vi "value to ring (PortType).vi"(11 "value":string) -> (3 "PortType":enum16{"FDX_UDP_SAMPLING", "FDX_UDP_QUEUING"}(ring))   [LabVIEW 2020, in "AIM ARINC 664 Import.lvlib"]
uses:
  AIM ARINC 664 Import.lvlib
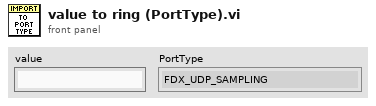
[diagram p1: front panel]
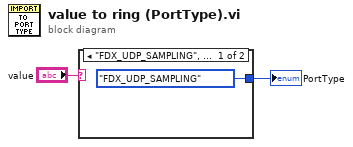
[diagram p0: block diagram]
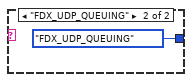
[diagram p2: hidden frame]
diagram:
  n1 = case shown="\"FDX_UDP_SAMPLING\", Default" "value" {
    tunnel: [enum16{"FDX_UDP_SAMPLING", "FDX_UDP_QUEUING"}."FDX_UDP_SAMPLING" ("PortType") enum16{"FDX_UDP_SAMPLING", "FDX_UDP_QUEUING"}."FDX_UDP_QUEUING" ("PortType")] -> w2
    frame "FDX_UDP_SAMPLING", Default {
    }
    frame "FDX_UDP_QUEUING" {
    }
  }
  "PortType" <- w2
